vi "FGV FT-IR Kalibrieren.vi"(10 "Aktionen FT-IR Kalibrieren":T1) -> (1 "Zustand FT-IR":string, 2 "Aktionen FT-IR Kalibrieren":T1)   [LabVIEW 2020, in "FT-IR.lvlib"]
uses:
  FT-IR.lvlib
  Aktionen FT-IR Kalibrieren.ctl
  FGV FT-IR Aktionen.ctl
  FGV FT-IR Gasliste Aktionen.ctl
  Sprachverwaltung/FGV Aktion Tabelle zerlegen.ctl
  Stoerungen/Stoerungen Messgeraet/Aktionen Kommunikation Stoerung.ctl
  SysLog/SysLog Interface.ctl
  Messdaten/Aktionen FGV Messdaten.ctl
  Schedule Modul/Aktion FGV Testdaten sammeln.ctl
  TOOLweb Interface Library/Trigger Aktionen.ctl
  Stoerungen/Stoerungen.lvlib
  Allgemein/allgemeine Sub-VIs.lvlib
  TOOLweb Interface Library/Typdefinitionen.lvlib
  TOOLweb Interface Library/TOOLweb Interface.lvlib
  Messdaten/Messdaten.lvlib
  Sprachverwaltung/Sprachverwaltung.lvlib
  SysLog/SysLog.lvlib
  Schedule Modul/Schedule Modul.lvlib
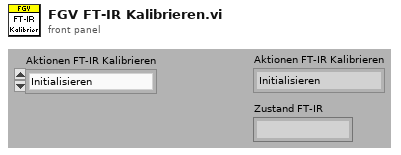
[diagram p1: front panel]
types:
  T1 = typedef "FT-IR.lvlib/Aktionen FT-IR Kalibrieren.ctl" = enum16{"Initialisieren", "Anstehende Störung", "CO2, H2O - Vergleichen", "Hintergrund starten", "Hintergrund", "Hintergrund Abgeschlossen", "Fertig", "Beenden"}
  T2 = typedef "Sprachverwaltung.lvlib/FGV Aktion Tabelle zerlegen.ctl" = enum16{"laden", "vereinzeln", "speichern"}
  T3 = typedef "FT-IR.lvlib/FGV FT-IR Gasliste Aktionen.ctl" = enum16{"lesen", "Gasliste FT-IR", "Gasliste ausgelesen", "laden", "speichern", "löschen"}
  T4 = typedef "FT-IR.lvlib/FGV FT-IR Aktionen.ctl" = enum16{"lesen", "NOG setzen", "NOS setzen", "Initialisieren", "speichern", "ALLES setzen", "FT-IR Spektrum loggen", "Komm Stoppen", "Spektrum LogKonfig"}
  T5 = typedef "Stoerungen.lvlib/Aktionen Kommunikation Stoerung.ctl" = enum16{"lesen", "init", "FT-IR Komm", "FT-IR Betriebsart", "FT-IR Hintergrund", "cRIO Komm", "PNS Komm", "Dichtheitstest", "Life Bit", "FTIR Komm AK", "PMA Komm", "FID Komm", "PMA Cal", "FID Ch4 Cal", "FID THC Cal", "Cal Timeout", "VFS 1 Komm", "VFS 2 Komm", "VFS 3 Komm", "VFS 4 Komm", "TRE 08 Komm", "CG-Test vorzeitig", "CG-Test Span 1", "CG-Test Span 2", "CG-Test Span 3", "CG-Test Messgas", "CG-Test löschen", "Test", "Amium AK", "AK Recept konfig", "AK Name konfig", "AK EKFG konfig"}
  T6 = typedef "SysLog.lvlib/SysLog Interface.ctl" = cluster{"FehlermeldungsCode":i32, "ErfolgsmeldungsCode":i32, "ParameterListenString":string, "Anzeige":bool, "SysLogIcon":enum16{"OK", "Warnung", "Fehler"}, "intern":bool}
  T7 = typedef "Messdaten.lvlib/Aktionen FGV Messdaten.ctl" = enum16{"lesen", "schreiben", "löschen", "Mittelwerte", "Komponente"}
  T8 = typedef "Schedule Modul.lvlib/Aktion FGV Testdaten sammeln.ctl" = enum16{"lesen", "Dichtheitstest", "CalGasTest", "T90", "Kalibrieren", "init", "Kalender Daten"}
  T9 = typedef "FT-IR.lvlib/TOOLweb Interface.lvlib/Typdefinitionen.lvlib/Trigger Aktionen.ctl" = enum16{"startrun", "runonce", "stoprun", "pauserun", "resumerun", "takeback"}
  T10 = typedef "String - Ausgabefeld.ctl" = string
  T11 = typedef "Stoerungen.lvlib/Stoerungen Messgeraete.ctl" = cluster{"FT-IR Komm":bool, "FT-IR Betriebsart":bool, "FT-IR Hintergrundscan":bool, "Dichtheitstest":bool, "cRIO Komm":bool, "PNS Komm":bool, "Life Bit":bool, "FT-IR AK Komm":bool, "PMA Komm":bool, "FID Komm":bool, "PMA Cal":bool, "FID CH4 Cal":bool, "FID THC Cal":bool, "Cal Timeout":bool, "VFS 1 Komm":bool, "VFS 2 Komm":bool, "VFS 3 Komm":bool, "VFS 4 Komm":bool, "TRE 08 Komm":bool, "CG-Test":bool, "CG-Test 1":bool, "CG-Test 2":bool, "CG-Test 3":bool, "Messgas - Eingang":bool, "Amium AK Komm":bool, "AK Rezept nicht konfiguriert ":bool, "AK Name nicht konfiguriert":bool, "AK EKFG nicht konfiguriert":bool}
  T12 = typedef "Schedule Modul.lvlib/Ergebnis Kalibrieren.ctl" = cluster{"Fehler":bool, "CO2 H2O vergleich":bool}
  T13 = typedef "FT-IR.lvlib/TOOLweb Interface.lvlib/Typdefinitionen.lvlib/TOOLweb Einstellungen.ctl" = cluster{"(1) InstrumentState":string, "(10) NrOfGasses":i32, "(21) recipeCurrent":string, "(80) labEnabled":bool, "(81) labPath":path, "(82) labBaseName":string, "(83) labIndex":string, "(90) ftirScans":i32}
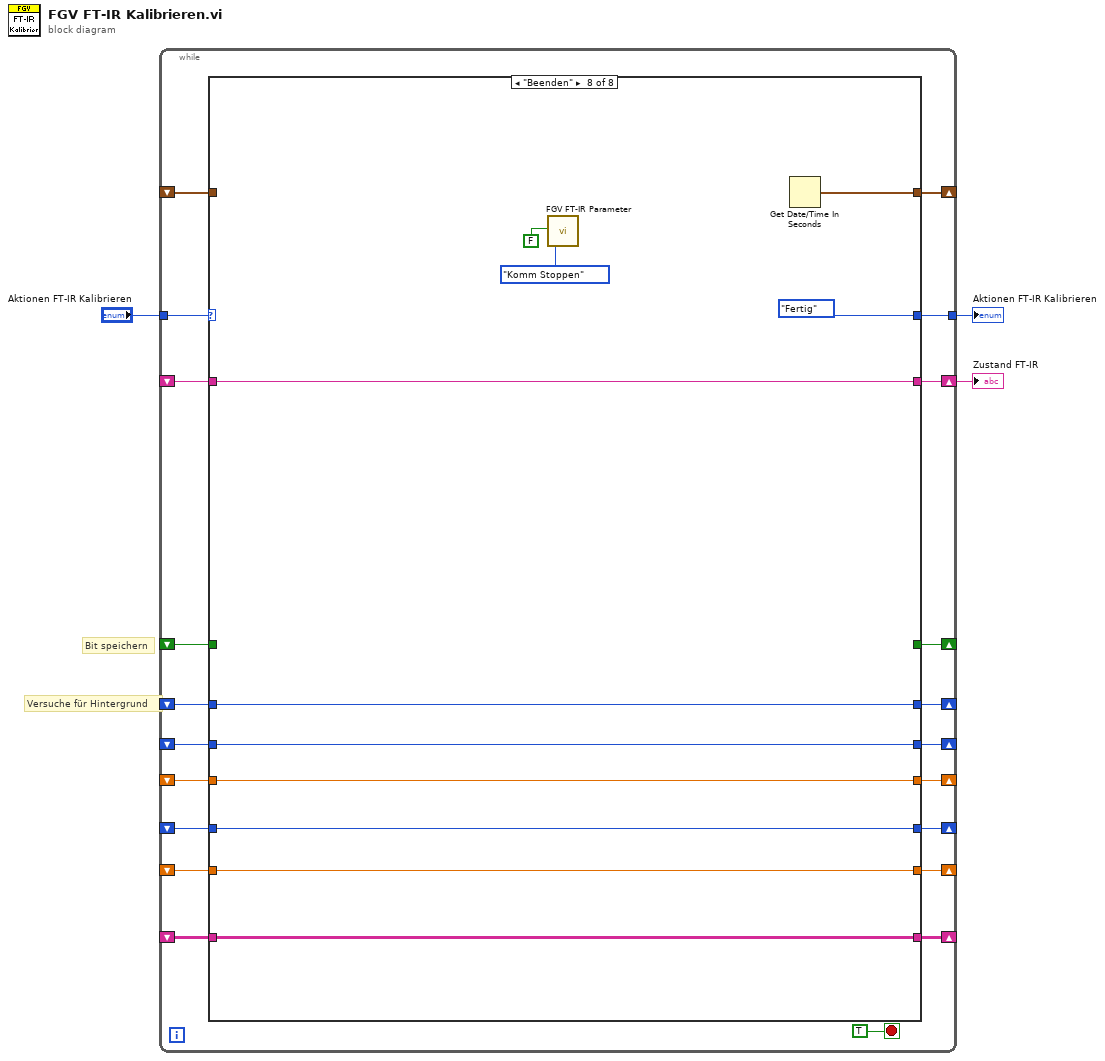
[diagram p0: block diagram]
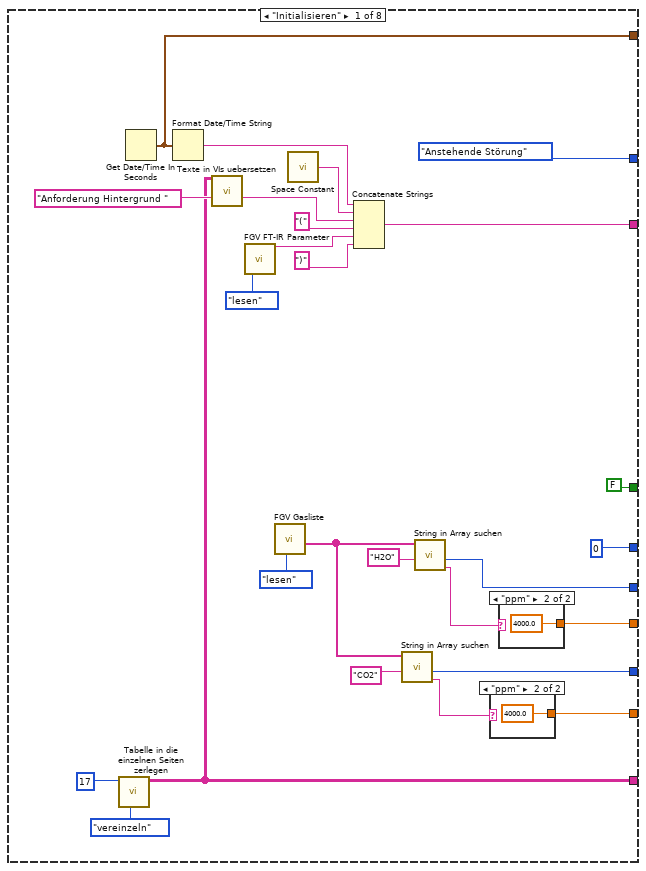
[diagram p2: hidden frame]
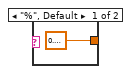
[diagram p3: hidden frame]
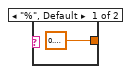
[diagram p4: hidden frame]
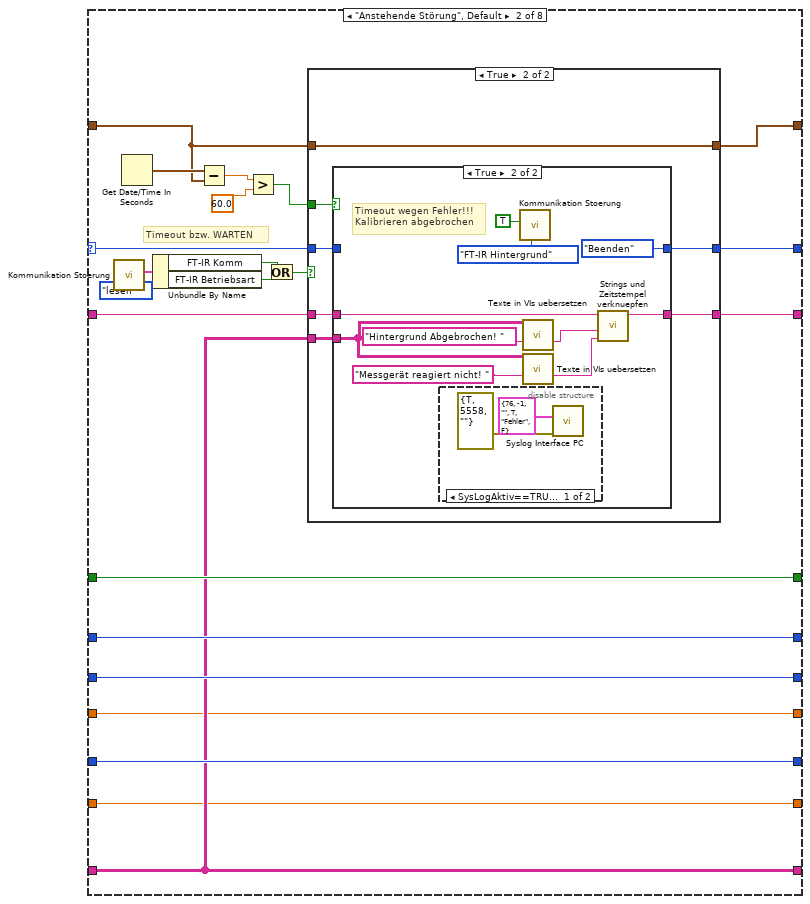
[diagram p5: hidden frame]
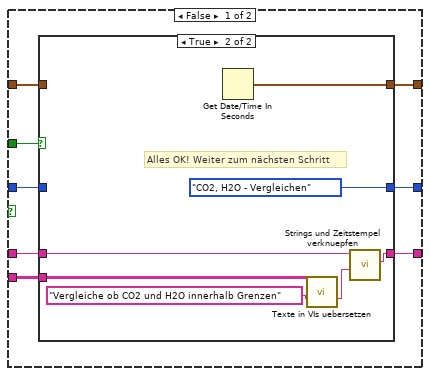
[diagram p6: hidden frame]
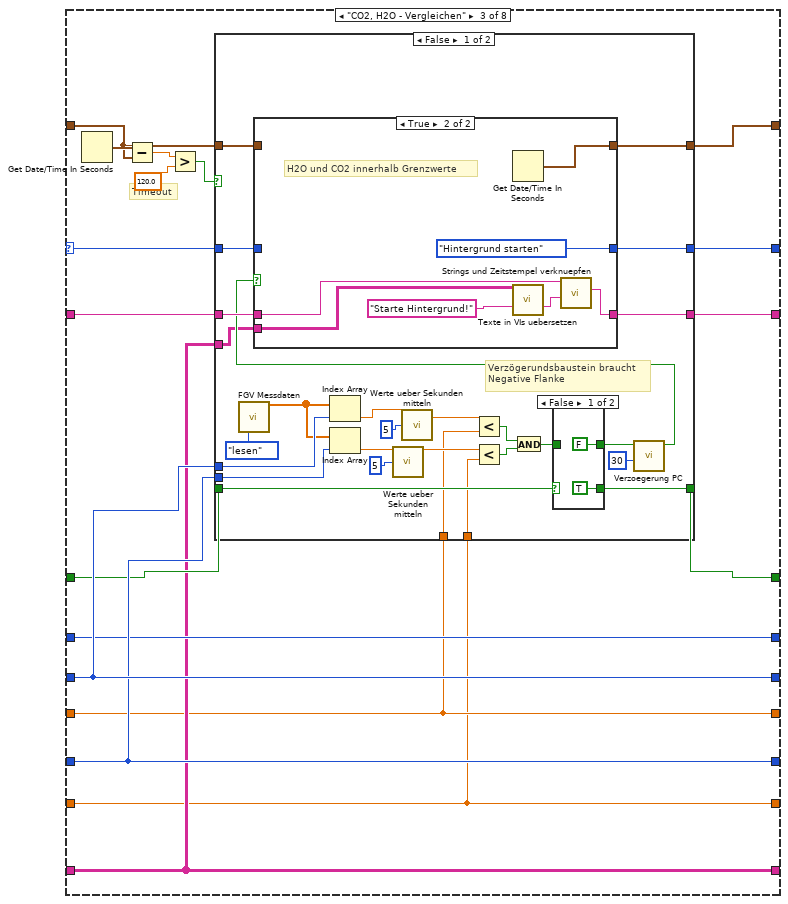
[diagram p10: hidden frame]
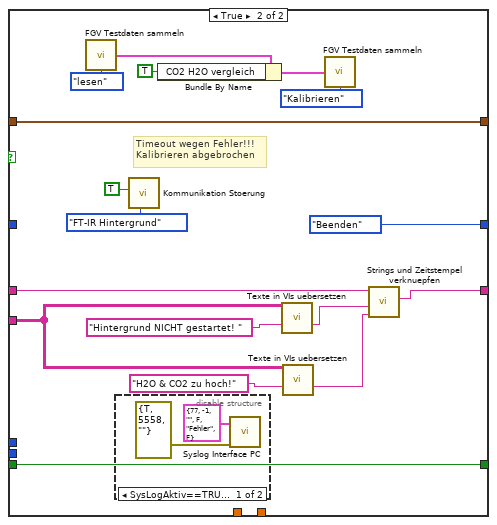
[diagram p13: hidden frame]
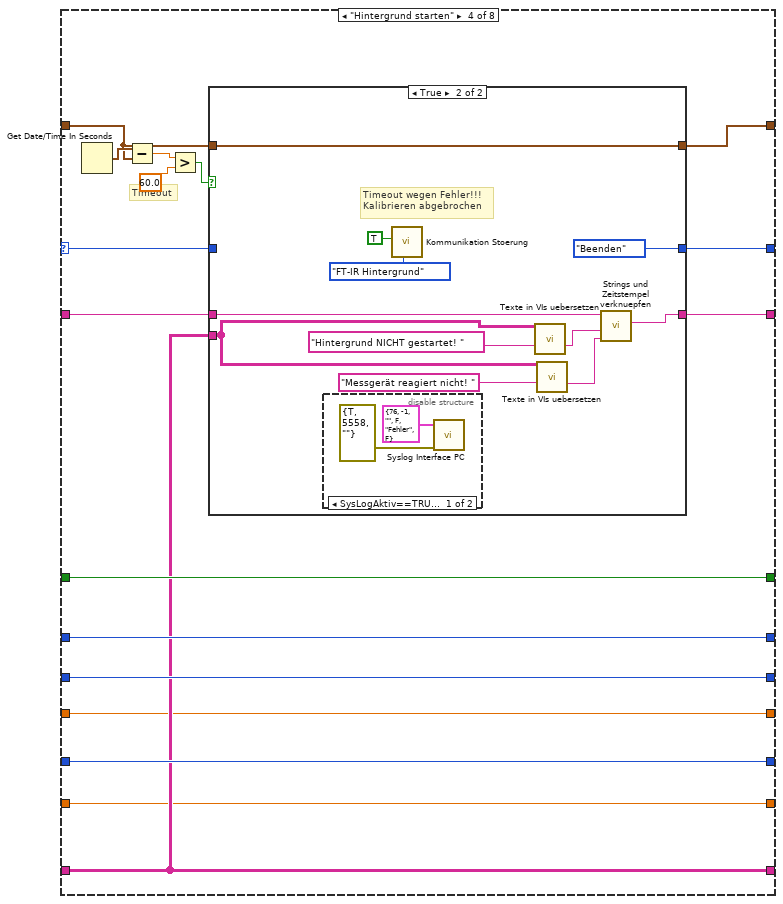
[diagram p15: hidden frame]
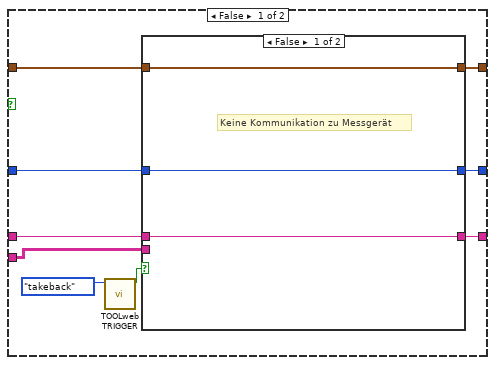
[diagram p16: hidden frame]
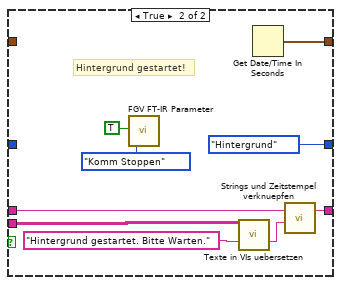
[diagram p17: hidden frame]
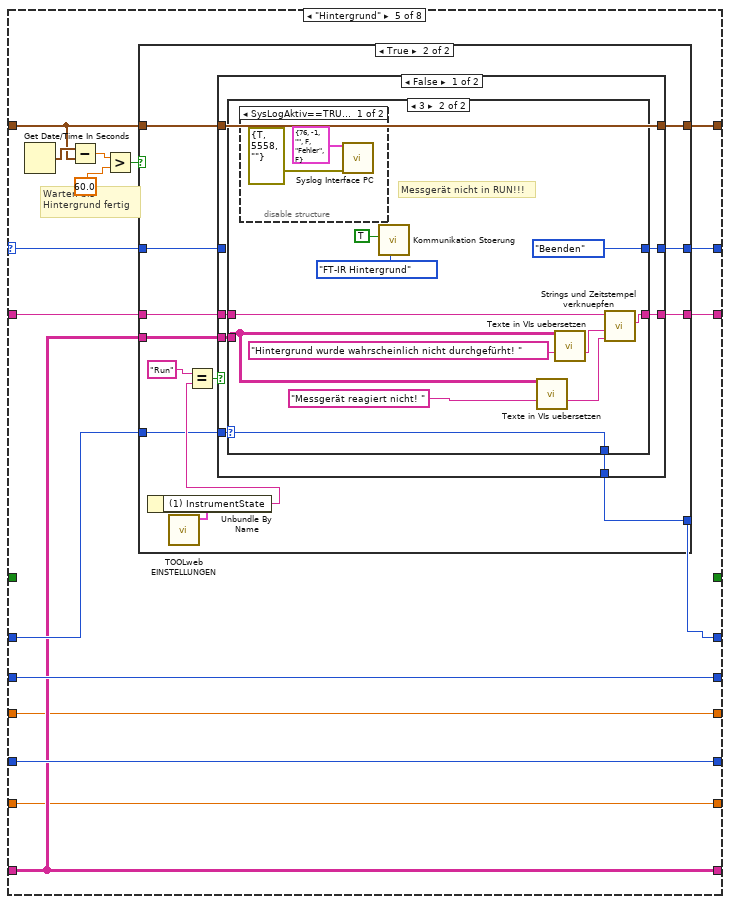
[diagram p19: hidden frame]
diagram:
  # "Versuche für Hintergrund"
  # "Bit speichern"
  n1 = while {
    shift-right: [w22] -> _
    shift-left: _ -> [w23]
    shift-right: [w18] -> w3
    shift-left: _ -> [w17]
    shift-right: [w15] -> _
    shift-left: _ -> [w20]
    shift-right: [w16] -> _
    shift-left: _ -> [w19]
    tunnel: "Aktionen FT-IR Kalibrieren" -> [w24]
    tunnel: [w21] -> w2
    shift-right: [w12] -> _
    shift-left: _ -> [w13]
    shift-right: [w11] -> _
    shift-left: _ -> [w10]
    shift-right: [w9] -> _
    shift-left: _ -> [w8]
    shift-right: [w7] -> _
    shift-left: _ -> [w6]
    shift-right: [w5] -> _
    shift-left: _ -> [w4]
    stop <- TRUE stop-if-true
    n2 = case shown="\"Beenden\"" w24 {
      selector: w24 -> [_ w70 w124 w201 w252 _ w347 _]
      tunnel: w23 -> [_ w66 w126 w202 w255 w338 w348 _]
      tunnel: [w43 w65 w125 w203 w254 w338 w348 w356] -> w22
      tunnel: [Aktionen_FT-IR_Kalibrieren."Anstehende Störung" ("Aktionen FT-IR Kalibrieren") w71 w129 w206 w256 Aktionen_FT-IR_Kalibrieren."Fertig" ("Aktionen FT-IR Kalibrieren") w347 Aktionen_FT-IR_Kalibrieren."Fertig" ("Aktionen FT-IR Kalibrieren")] -> w21
      tunnel: w17 -> [_ w68 w128 w205 w257 w337 w346 w354]
      tunnel: [w42 w67 w127 w204 w253 w336 w346 w354] -> w18
      tunnel: w20 -> [_ w64 w123 w200 w251 w335 w345 w359]
      tunnel: w19 -> [_ w63 w122 w199 w250 w334 w344 w358]
      tunnel: [w37 w63 w122 w199 w250 w334 w344 w358] -> w16
      tunnel: [w38 w64 w123 w200 w251 w335 w345 w359] -> w15
      tunnel: w13 -> [_ w58 w121 w197 _ _ _ _]
      tunnel: [FALSE w58 w120 w197 _ _ _ _] -> w12
      tunnel: [u16 0 w59 w119 w198 w248 w333 w343 w355] -> w11
      tunnel: w10 -> [_ w59 w119 w198 w249 w333 w343 w355]
      tunnel: [w30 w57 w118 w196 w247 w328 w342 w351] -> w9
      tunnel: w8 -> [_ w57 w118 w196 w247 w328 w342 w351]
      tunnel: [w26 w56 w116 w195 w246 w327 w341 w350] -> w7
      tunnel: w6 -> [_ w56 w116 w195 w246 w327 w341 w350]
      tunnel: [w25 w55 w117 w194 w245 w326 w340 w349] -> w5
      tunnel: w4 -> [_ w55 w117 w194 w245 w326 w340 w349]
      frame "Initialisieren" {
        n3 = call "Tabelle in die einzelnen Seiten zerlegen.vi"("Aktion"=FGV_Aktion_Tabelle_zerlegen."vereinzeln", "Index (Seite)"=17) -> ("Sprachliste"=w30:string[][])  [unwired: 7 in, 2 out]
        n4 = Get Date/Time In Seconds() -> (seconds since 1Jan1904=w43:timestamp)
        n5 = Format Date/Time String(seconds (now)=w43) -> (date/time string=w44:string)  [unwired: 2 in]
        n6 = call "Texte in VIs uebersetzen.vi"("Sprachliste"=w30, "String zum Übersetzen"="Anforderung Hintergrund " ("String")) -> ("String zum Übersetzen"=w32:string)  [unwired: 9 in, 4 out]
        n7 = call "FGV FT-IR Parameter.vi"("Aktion"=FGV_FT-IR_Aktionen."lesen") -> ("Instrument State"=w47:string)  [unwired: 11 in, 7 out]
        n8 = call "FGV Gasliste.vi"("Aktionen"=FGV_FT-IR_Gasliste_Aktionen."lesen") -> ("Aktuelle Gasliste gesamt"=w35:T10[])  [unwired: 8 in, 2 out]
        n9 = call <vilib>:"Space Constant.vi"() -> ("String"=w49:string)
        n10 = Concatenate Strings(w44, w49, w32, "(" ("String"), w47, ")" ("String")) -> (w42:string)
        n11 = call "String in Array suchen.vi"("Nach String/Zeichen suchen (-)"="CO2", "String-Array"=w35) -> ("Einheit"=w27:string, "Index"=w37:i32)  [unwired: 7 in, 1 out]
        n12 = call "String in Array suchen.vi"("Nach String/Zeichen suchen (-)"="H2O", "String-Array"=w35) -> ("Einheit"=w28:string, "Index"=w38:i32)  [unwired: 7 in, 1 out]
        n13 = case shown="\"ppm\"" w27 {
          tunnel: [sgl 0.4 ("y") sgl 4000.0 ("y")] -> w26
          frame "%", Default {
          }
          frame "ppm" {
          }
        }
        n14 = case shown="\"ppm\"" w28 {
          tunnel: [sgl 0.4 ("y") sgl 4000.0 ("y")] -> w25
          frame "%", Default {
          }
          frame "ppm" {
          }
        }
      }
      frame "Anstehende Störung", Default {
        # "Timeout bzw. WARTEN"
        n15 = call "Kommunikation Stoerung.vi"("Aktionen"=Aktionen_Kommunikation_Stoerung."lesen") -> ("Störung Messgerät"=w75:T11)  [unwired: 2 in, 8 out]
        n16 = Get Date/Time In Seconds() -> (seconds since 1Jan1904=w74:timestamp)
        n17 = Unbundle By Name(w75) -> ("FT-IR Komm"=w62:bool, "FT-IR Betriebsart"=w61:bool)
        n18 = Subtract(x=w74, y=w66) -> (x-y=w73:dbl)
        n19 = Greater?(x=w73, y=60.0) -> (0:w69:bool)
        n20 = Or(x=w62, y=w61) -> (x .or. y?=w60:bool)
        n21 = case shown="True" w60 {
          tunnel: [w84 w99] -> w71
          tunnel: w70 -> [w79 w100]
          tunnel: w69 -> [w80 w101]
          tunnel: w68 -> [w82 w98]
          tunnel: [w81 w97] -> w67
          tunnel: w66 -> [w78 w96]
          tunnel: [w83 w96] -> w65
          tunnel: w57 -> [w77 w95]
          frame False {
            n22 = case shown="True" w80 {
              tunnel: [w87 Aktionen_FT-IR_Kalibrieren."CO2, H2O - Vergleichen" ("Aktionen FT-IR Kalibrieren")] -> w84
              tunnel: [w86 w93] -> w83
              tunnel: w82 -> [w85 w92]
              tunnel: [w85 w91] -> w81
              tunnel: w79 -> [w87 _]
              tunnel: w78 -> [w86 _]
              tunnel: w77 -> [_ w88]
              frame False {
                # "Warten bis Messzelle gespült!"
              }
              frame True {
                # "Alles OK! Weiter zum nächsten Schritt"
                n23 = Get Date/Time In Seconds() -> (seconds since 1Jan1904=w93:timestamp)
                n24 = call "Texte in VIs uebersetzen.vi"("Sprachliste"=w88, "String zum Übersetzen"="Vergleiche ob CO2 und H2O innerhalb Grenzen" ("String")) -> ("String zum Übersetzen"=w89:string)  [unwired: 9 in, 4 out]
                n25 = call "Strings und Zeitstempel verknuepfen.vi"("String 1 hinzufügen"=w89, "Eingagns String"=w92) -> ("Verknüpfter String"=w91:string)  [unwired: 9 in]
              }
            }
          }
          frame True {
            n26 = case shown="True" w101 {
              tunnel: w100 -> [w103 _]
              tunnel: [w103 Aktionen_FT-IR_Kalibrieren."Beenden" ("Aktionen FT-IR Kalibrieren")] -> w99
              tunnel: w98 -> [w102 w112]
              tunnel: [w102 w111] -> w97
              tunnel: w95 -> [_ w104]
              frame False {
                # "Fehler steht an!!!!"
              }
              frame True {
                # "Timeout wegen Fehler!!! \nKalibrieren abgebrochen"
                n27 = disable-structure shown="SysLogAktiv==TRUE, Standard" {
                  frame condition #0 (active) {
                    n28 = call "Syslog Interface PC.vi"("Fehler (in)"=errorcluster {"status"=TRUE, "code"=5558, "source"=""}, "Cluster (in)"=T6 {"FehlermeldungsCode"=76, "ErfolgsmeldungsCode"=-1, "ParameterListenString"="", "Anzeige"=TRUE, "SysLogIcon"=enum."Fehler", "intern"=FALSE}) -> ()  [unwired: 9 in, 1 out]
                  }
                  frame condition #1 {
                  }
                }
                n29 = call "Kommunikation Stoerung.vi"("Aktionen"=Aktionen_Kommunikation_Stoerung."FT-IR Hintergrund", "ERROR"=TRUE) -> ()  [unwired: 9 in, 1 out]
                n30 = call "Texte in VIs uebersetzen.vi"("Sprachliste"=w104, "String zum Übersetzen"="Hintergrund Abgebrochen! " ("String")) -> ("String zum Übersetzen"=w107:string)  [unwired: 9 in, 4 out]
                n31 = call "Texte in VIs uebersetzen.vi"("Sprachliste"=w104, "String zum Übersetzen"="Messgerät reagiert nicht! " ("String")) -> ("String zum Übersetzen"=w105:string)  [unwired: 9 in, 4 out]
                n32 = call "Strings und Zeitstempel verknuepfen.vi"("String 2 hinzufügen"=w105, "String 1 hinzufügen"=w107, "Eingagns String"=w112) -> ("Verknüpfter String"=w111:string)  [unwired: 8 in]
              }
            }
          }
        }
      }
      frame "CO2, H2O - Vergleichen" {
        # "Timeout"
        n33 = Get Date/Time In Seconds() -> (seconds since 1Jan1904=w133:timestamp)
        n34 = Subtract(x=w133, y=w126) -> (x-y=w132:dbl)
        n35 = Greater?(x=w132, y=120.0) -> (0:w130:bool)
        n36 = case shown="False" w130 {
          tunnel: [w156 Aktionen_FT-IR_Kalibrieren."Beenden" ("Aktionen FT-IR Kalibrieren")] -> w129
          tunnel: w128 -> [w158 w190]
          tunnel: [w157 w189] -> w127
          tunnel: w122 -> [w160 _]
          tunnel: w123 -> [w159 _]
          tunnel: w126 -> [w154 w175]
          tunnel: [w153 w175] -> w125
          tunnel: w124 -> [w155 _]
          tunnel: w121 -> [w148 w188]
          tunnel: [w147 w188] -> w120
          tunnel: w118 -> [w136 w181]
          tunnel: w117 -> [w135 _]
          tunnel: w116 -> [w134 _]
          frame False {
            # "Verzögerundsbaustein braucht\nNegative Flanke"
            n37 = call "FGV Messdaten.vi"("Aktionen"=Aktionen_FGV_Messdaten."lesen") -> ("Aktuelle Messwerte"=w145:sgl[])  [unwired: 6 in, 8 out]
            n38 = Index Array(array=w145, index=w159) -> (element=w142:sgl)
            n39 = Index Array(array=w145, index=w160) -> (element=w140:sgl)
            n40 = call "Werte ueber Sekunden mitteln.vi"("Neuer Wert"=w140, "Sek"=u8 5 ("Anzahl Werte")) -> ("gemittelter Wert"=w139:sgl)  [unwired: 12 in, 1 out]
            n41 = call "Werte ueber Sekunden mitteln.vi"("Neuer Wert"=w142, "Sek"=u8 5 ("Anzahl Werte")) -> ("gemittelter Wert"=w141:sgl)  [unwired: 12 in, 1 out]
            n42 = Less?(x=w141, y=w135) -> (x < y?=w144:bool)
            n43 = Less?(x=w139, y=w134) -> (x < y?=w143:bool)
            n44 = And(x=w144, y=w143) -> (x .and. y?=w150:bool)
            n45 = case shown="False" w148 {
              selector: w148 -> [_ w164]
              tunnel: w150 -> [_ w163]
              tunnel: [FALSE w163] -> w149
              tunnel: [TRUE w164] -> w147
              frame False {
              }
              frame True {
              }
            }
            n46 = call "Verzoegerung PC.vi"("sec"=u16 30, "Startsignal"=w149) -> ("Zeit abgelaufen?"=w151:bool)  [unwired: 8 in, 1 out]
            n47 = case shown="True" w151 {
              tunnel: w158 -> [w167 w172]
              tunnel: [w167 w171] -> w157
              tunnel: [w166 Aktionen_FT-IR_Kalibrieren."Hintergrund starten" ("Aktionen FT-IR Kalibrieren")] -> w156
              tunnel: w155 -> [w166 _]
              tunnel: w154 -> [w165 _]
              tunnel: [w165 w173] -> w153
              tunnel: w136 -> [_ w168]
              frame False {
                # "H2O und CO2 NICHT innerhalb Grenzwerte"
              }
              frame True {
                # "H2O und CO2 innerhalb Grenzwerte"
                n48 = Get Date/Time In Seconds() -> (seconds since 1Jan1904=w173:timestamp)
                n49 = call "Texte in VIs uebersetzen.vi"("Sprachliste"=w168, "String zum Übersetzen"="Starte Hintergrund!" ("String")) -> ("String zum Übersetzen"=w169:string)  [unwired: 9 in, 4 out]
                n50 = call "Strings und Zeitstempel verknuepfen.vi"("String 1 hinzufügen"=w169, "Eingagns String"=w172) -> ("Verknüpfter String"=w171:string)  [unwired: 9 in]
              }
            }
          }
          frame True {
            # "Timeout wegen Fehler!!! \nKalibrieren abgebrochen"
            n51 = call "FGV Testdaten sammeln.vi"("Aktion"=Aktion_FGV_Testdaten_sammeln."lesen") -> ("Ergebnisse Kalibrieren"=w178:T12)  [unwired: 9 in, 5 out]
            n52 = disable-structure shown="SysLogAktiv==TRUE" {
              frame condition #0 (active) {
                n53 = call "Syslog Interface PC.vi"("Fehler (in)"=errorcluster {"status"=TRUE, "code"=5558, "source"=""}, "Cluster (in)"=T6 {"FehlermeldungsCode"=77, "ErfolgsmeldungsCode"=-1, "ParameterListenString"="", "Anzeige"=FALSE, "SysLogIcon"=enum."Fehler", "intern"=FALSE}) -> ()  [unwired: 9 in, 1 out]
              }
              frame condition #1 {
              }
            }
            n54 = call "Kommunikation Stoerung.vi"("Aktionen"=Aktionen_Kommunikation_Stoerung."FT-IR Hintergrund", "ERROR"=TRUE) -> ()  [unwired: 9 in, 1 out]
            n55 = Bundle By Name(cluster=w178, "CO2 H2O vergleich"=TRUE) -> (w176:T12)
            n56 = call "Texte in VIs uebersetzen.vi"("Sprachliste"=w181, "String zum Übersetzen"="Hintergrund NICHT gestartet! " ("String")) -> ("String zum Übersetzen"=w184:string)  [unwired: 9 in, 4 out]
            n57 = call "Texte in VIs uebersetzen.vi"("Sprachliste"=w181, "String zum Übersetzen"="H2O & CO2 zu hoch!" ("String")) -> ("String zum Übersetzen"=w182:string)  [unwired: 9 in, 4 out]
            n58 = call "FGV Testdaten sammeln.vi"("Ergebnisse Kalibrieren"=w176, "Aktion"=Aktion_FGV_Testdaten_sammeln."Kalibrieren") -> ()  [unwired: 8 in, 6 out]
            n59 = call "Strings und Zeitstempel verknuepfen.vi"("String 2 hinzufügen"=w182, "String 1 hinzufügen"=w184, "Eingagns String"=w190) -> ("Verknüpfter String"=w189:string)  [unwired: 8 in]
          }
        }
      }
      frame "Hintergrund starten" {
        # "Timeout"
        n60 = Get Date/Time In Seconds() -> (seconds since 1Jan1904=w210:timestamp)
        n61 = Subtract(x=w210, y=w202) -> (x-y=w209:dbl)
        n62 = Greater?(x=w209, y=60.0) -> (0:w207:bool)
        n63 = case shown="True" w207 {
          tunnel: [w218 Aktionen_FT-IR_Kalibrieren."Beenden" ("Aktionen FT-IR Kalibrieren")] -> w206
          tunnel: w205 -> [w217 w240]
          tunnel: [w214 w239] -> w204
          tunnel: [w215 w241] -> w203
          tunnel: w202 -> [w216 w241]
          tunnel: w201 -> [w219 _]
          tunnel: w196 -> [w211 w232]
          frame False {
            n64 = call "TOOLweb TRIGGER.vi"("action"=Trigger_Aktionen."takeback") -> ("Trigger ausgeführt"=w212:bool)  [unwired: 5 in, 1 out]
            n65 = case shown="False" w212 {
              tunnel: w219 -> [w222 _]
              tunnel: [w222 Aktionen_FT-IR_Kalibrieren."Hintergrund" ("Aktionen FT-IR Kalibrieren")] -> w218
              tunnel: w217 -> [w221 w231]
              tunnel: w216 -> [w220 _]
              tunnel: [w220 w228] -> w215
              tunnel: [w221 w230] -> w214
              tunnel: w211 -> [_ w223]
              frame False {
                # "Keine Kommunikation zu Messgerät"
              }
              frame True {
                # "Hintergrund gestartet!"
                n66 = call "FGV FT-IR Parameter.vi"("Komm Stoppen"=TRUE, "Aktion"=FGV_FT-IR_Aktionen."Komm Stoppen") -> ()  [unwired: 10 in, 8 out]
                n67 = call "Texte in VIs uebersetzen.vi"("Sprachliste"=w223, "String zum Übersetzen"="Hintergrund gestartet. Bitte Warten." ("String")) -> ("String zum Übersetzen"=w224:string)  [unwired: 9 in, 4 out]
                n68 = Get Date/Time In Seconds() -> (seconds since 1Jan1904=w228:timestamp)
                n69 = call "Strings und Zeitstempel verknuepfen.vi"("String 1 hinzufügen"=w224, "Eingagns String"=w231) -> ("Verknüpfter String"=w230:string)  [unwired: 9 in]
              }
            }
          }
          frame True {
            # "Timeout wegen Fehler!!! \nKalibrieren abgebrochen"
            n70 = disable-structure shown="SysLogAktiv==TRUE" {
              frame condition #0 (active) {
                n71 = call "Syslog Interface PC.vi"("Fehler (in)"=errorcluster {"status"=TRUE, "code"=5558, "source"=""}, "Cluster (in)"=T6 {"FehlermeldungsCode"=76, "ErfolgsmeldungsCode"=-1, "ParameterListenString"="", "Anzeige"=FALSE, "SysLogIcon"=enum."Fehler", "intern"=FALSE}) -> ()  [unwired: 9 in, 1 out]
              }
              frame condition #1 {
              }
            }
            n72 = call "Kommunikation Stoerung.vi"("Aktionen"=Aktionen_Kommunikation_Stoerung."FT-IR Hintergrund", "ERROR"=TRUE) -> ()  [unwired: 9 in, 1 out]
            n73 = call "Texte in VIs uebersetzen.vi"("Sprachliste"=w232, "String zum Übersetzen"="Hintergrund NICHT gestartet! " ("String")) -> ("String zum Übersetzen"=w235:string)  [unwired: 9 in, 4 out]
            n74 = call "Texte in VIs uebersetzen.vi"("Sprachliste"=w232, "String zum Übersetzen"="Messgerät reagiert nicht! " ("String")) -> ("String zum Übersetzen"=w233:string)  [unwired: 9 in, 4 out]
            n75 = call "Strings und Zeitstempel verknuepfen.vi"("String 2 hinzufügen"=w233, "String 1 hinzufügen"=w235, "Eingagns String"=w240) -> ("Verknüpfter String"=w239:string)  [unwired: 8 in]
          }
        }
      }
      frame "Hintergrund" {
        # "Warten bis \nHintergrund fertig"
        n76 = Get Date/Time In Seconds() -> (seconds since 1Jan1904=w261:timestamp)
        n77 = Subtract(x=w261, y=w255) -> (x-y=w260:dbl)
        n78 = Greater?(x=w260, y=60.0) -> (0:w258:bool)
        n79 = case shown="True" w258 {
          tunnel: w257 -> [w263 w274]
          tunnel: [w264 w275] -> w256
          tunnel: w255 -> [w265 w277]
          tunnel: [w265 w276] -> w254
          tunnel: [w263 w273] -> w253
          tunnel: w252 -> [w264 w272]
          tunnel: w249 -> [w262 w267]
          tunnel: [w262 w270] -> w248
          tunnel: w247 -> [_ w266]
          frame False {
          }
          frame True {
            n80 = call "TOOLweb EINSTELLUNGEN.vi"() -> ("Einstellungen"=w269:T13)  [unwired: 7 in]
            n81 = Unbundle By Name(w269) -> ("(1) InstrumentState"=w268:string)
            n82 = Equal?(x="Run", y=w268) -> (x = y?=w271:bool)
            n83 = case shown="False" w271 {
              tunnel: w277 -> [w285 _]
              tunnel: [w285 w325] -> w276
              tunnel: [w284 Aktionen_FT-IR_Kalibrieren."Hintergrund Abgeschlossen" ("Aktionen FT-IR Kalibrieren")] -> w275
              tunnel: w274 -> [w282 w323]
              tunnel: [w283 w322] -> w273
              tunnel: w272 -> [_ _]
              tunnel: [w281 w321] -> w270
              tunnel: w267 -> [w280 w321]
              tunnel: w266 -> [w279 w316]
              frame False {
                n84 = case shown="3" w280 {
                  selector: w280 -> [w299 w308]
                  tunnel: [w292 Aktionen_FT-IR_Kalibrieren."Beenden" ("Aktionen FT-IR Kalibrieren")] -> w284
                  tunnel: [w293 w312] -> w283
                  tunnel: w282 -> [w294 w311]
                  tunnel: [w295 w308] -> w281
                  tunnel: w279 -> [w286 w303]
                  frame 0, Default {
                    n85 = flat-sequence {
                      tunnel: [Aktionen_FT-IR_Kalibrieren."Hintergrund starten" ("Aktionen FT-IR Kalibrieren")] -> w292
                      frame #0 {
                        n86 = call "TOOLweb TRIGGER.vi"("action"=Trigger_Aktionen."startrun") -> ()  [unwired: 5 in, 2 out]
                      }
                      frame #1 {
                        n87 = Wait (ms)(milliseconds to wait=u32 10000 ("Zu wartende ms")) -> ()  [unwired: 1 out]
                      }
                    }
                    n88 = Increment(x=w299) -> (x+1=w295:u16)
                    n89 = call "Texte in VIs uebersetzen.vi"("Sprachliste"=w286, "String zum Übersetzen"="Starte neuen Versuch" ("String")) -> ("String zum Übersetzen"=w289:string)  [unwired: 9 in, 4 out]
                    n90 = Number To Decimal String(number=w295) -> (decimal integer string=w298:string)  [unwired: 1 in]
                    n91 = Concatenate Strings(w289, "(" ("String"), w298, ")" ("String")) -> (w296:string)
                    n92 = call "Texte in VIs uebersetzen.vi"("Sprachliste"=w286, "String zum Übersetzen"="Hintergrund wurde wahrscheinlich nicht durchgefürht! " ("String")) -> ("String zum Übersetzen"=w287:string)  [unwired: 9 in, 4 out]
                    n93 = call "Strings und Zeitstempel verknuepfen.vi"("String 2 hinzufügen"=w296, "String 1 hinzufügen"=w287, "Eingagns String"=w294) -> ("Verknüpfter String"=w293:string)  [unwired: 8 in]
                  }
                  frame 3 {
                    # "Messgerät nicht in RUN!!!"
                    n94 = disable-structure shown="SysLogAktiv==TRUE" {
                      frame condition #0 (active) {
                        n95 = call "Syslog Interface PC.vi"("Fehler (in)"=errorcluster {"status"=TRUE, "code"=5558, "source"=""}, "Cluster (in)"=T6 {"FehlermeldungsCode"=76, "ErfolgsmeldungsCode"=-1, "ParameterListenString"="", "Anzeige"=FALSE, "SysLogIcon"=enum."Fehler", "intern"=FALSE}) -> ()  [unwired: 9 in, 1 out]
                      }
                      frame condition #1 {
                      }
                    }
                    n96 = call "Kommunikation Stoerung.vi"("Aktionen"=Aktionen_Kommunikation_Stoerung."FT-IR Hintergrund", "ERROR"=TRUE) -> ()  [unwired: 9 in, 1 out]
                    n97 = call "Texte in VIs uebersetzen.vi"("Sprachliste"=w303, "String zum Übersetzen"="Messgerät reagiert nicht! " ("String")) -> ("String zum Übersetzen"=w304:string)  [unwired: 9 in, 4 out]
                    n98 = call "Texte in VIs uebersetzen.vi"("Sprachliste"=w303, "String zum Übersetzen"="Hintergrund wurde wahrscheinlich nicht durchgefürht! " ("String")) -> ("String zum Übersetzen"=w306:string)  [unwired: 9 in, 4 out]
                    n99 = call "Strings und Zeitstempel verknuepfen.vi"("String 2 hinzufügen"=w304, "String 1 hinzufügen"=w306, "Eingagns String"=w311) -> ("Verknüpfter String"=w312:string)  [unwired: 8 in]
                  }
                }
              }
              frame True {
                n100 = call "FGV FT-IR Parameter.vi"("Komm Stoppen"=FALSE, "Aktion"=FGV_FT-IR_Aktionen."Komm Stoppen") -> ()  [unwired: 10 in, 8 out]
                n101 = call "Texte in VIs uebersetzen.vi"("Sprachliste"=w316, "String zum Übersetzen"="Hintergrund beendet." ("String")) -> ("String zum Übersetzen"=w317:string)  [unwired: 9 in, 4 out]
                n102 = call "Strings und Zeitstempel verknuepfen.vi"("String 1 hinzufügen"=w317, "Eingagns String"=w323) -> ("Verknüpfter String"=w322:string)  [unwired: 9 in]
                n103 = Get Date/Time In Seconds() -> (seconds since 1Jan1904=w325:timestamp)
              }
            }
          }
        }
      }
      frame "Hintergrund Abgeschlossen" {
        n104 = call "FGV FT-IR Parameter.vi"("Komm Stoppen"=FALSE, "Aktion"=FGV_FT-IR_Aktionen."Komm Stoppen") -> ()  [unwired: 10 in, 8 out]
        n105 = call "Texte in VIs uebersetzen.vi"("Sprachliste"=w328, "String zum Übersetzen"="Kalibrierung FT-IR abgeschlossen" ("String")) -> ("String zum Übersetzen"=w329:string)  [unwired: 9 in, 4 out]
        n106 = call "Strings und Zeitstempel verknuepfen.vi"("String 1 hinzufügen"=w329, "Eingagns String"=w337) -> ("Verknüpfter String"=w336:string)  [unwired: 9 in]
      }
      frame "Fertig" {
      }
      frame "Beenden" {
        n107 = call "FGV FT-IR Parameter.vi"("Komm Stoppen"=FALSE, "Aktion"=FGV_FT-IR_Aktionen."Komm Stoppen") -> ()  [unwired: 10 in, 8 out]
        n108 = Get Date/Time In Seconds() -> (seconds since 1Jan1904=w356:timestamp)
      }
    }
  }
  "Zustand FT-IR" <- w3
  "Aktionen FT-IR Kalibrieren" <- w2
